vi "pulse_generator_data_v3.vi"(3 "Pulse Generator Offsets & Data Saving Controls":T3={"PG-TS Offset"=11500.0, "Pitot Offset"=0.0, "PG Abs Offset"=11500.0, "Sampling\nFrequency"=1000.0, "Recording Duration"=10.0}, 4 "PG Data":waveform(dbl)[](array[waveform]), 5 "Session Start Time":timestamp) -> (0 "Pulse Generator Charts":T1={" Camera Voltage"=9.650720988784618, "Pitot dP"=-0.0006103608758678569, "Absolute Tank Pressure"=119484.80284900061, "Pulse Generator to Test Section dP"=11360.460004869077}, 1 "Pulse Generator Measurements":T2={"PG to TS dP"=4351.8068090218785, "PG Abs"=119484.80284900061, "Mass Flow Rate"=nan, "Pitot dP"=-4308.9404273994505, "Pitot Amps"=2.6415199999999147e-07, "Vapor Temperature"=19.805676371442082, "Liquid Temperature"=19.52526901660894, "Vapor Sat Pressure"=121.24568157832624, "Liquid Sat Pressure"=119.96937909943745, "W1-4 dP[Pa]"=19.52526901660894, "W1-7 dP[Pa]"=119.96937909943745}, 2 "PG Data - Queue":dbl[][](array[numeric]))   [LabVIEW 2016]
uses:
  Sensor Translation/sensor_translation.lvlib
  Sensor Translation/Pressure Transducers/Omega/omega_px209_060a5v.vi
  pulse_generator_data.ctl
  <vilib>/Waveform/WDTOps.llb/WDT Get Waveform Time Array DBL.vi
  pulse_generator_data_charts.ctl
  pulse_generator_data_controls.ctl
panel:
  # "Pulse Generator - Test Section dP"
  # "Pulse Generator Absolute Pressure"
  # "Pitot dP"
  # "Pitot Current"
  # "Mass Flow Rate"
  # "Offsets"
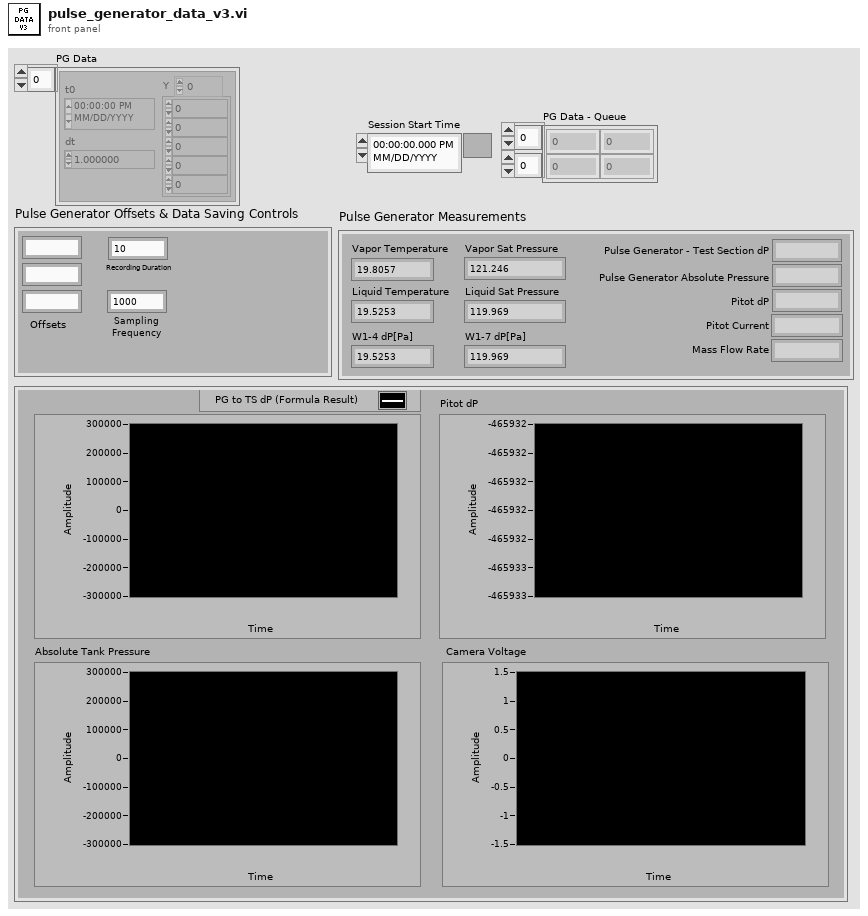
[diagram p1: front panel]
types:
  T1 = typedef "pulse_generator_data_charts.ctl" = cluster{" Camera Voltage":dbl, "Pitot dP":dbl, "Absolute Tank Pressure":dbl, "Pulse Generator to Test Section dP":dbl}
  T2 = typedef "pulse_generator_data.ctl" = cluster{"PG to TS dP":dbl, "PG Abs":dbl, "Mass Flow Rate":dbl, "Pitot dP":dbl, "Pitot Amps":dbl, "Vapor Temperature":dbl, "Liquid Temperature":dbl, "Vapor Sat Pressure":dbl, "Liquid Sat Pressure":dbl, "W1-4 dP[Pa]":dbl, "W1-7 dP[Pa]":dbl}
  T3 = typedef "pulse_generator_data_controls.ctl" = cluster{"PG-TS Offset":dbl, "Pitot Offset":dbl, "PG Abs Offset":dbl, "Sampling\nFrequency":dbl, "Recording Duration":dbl}
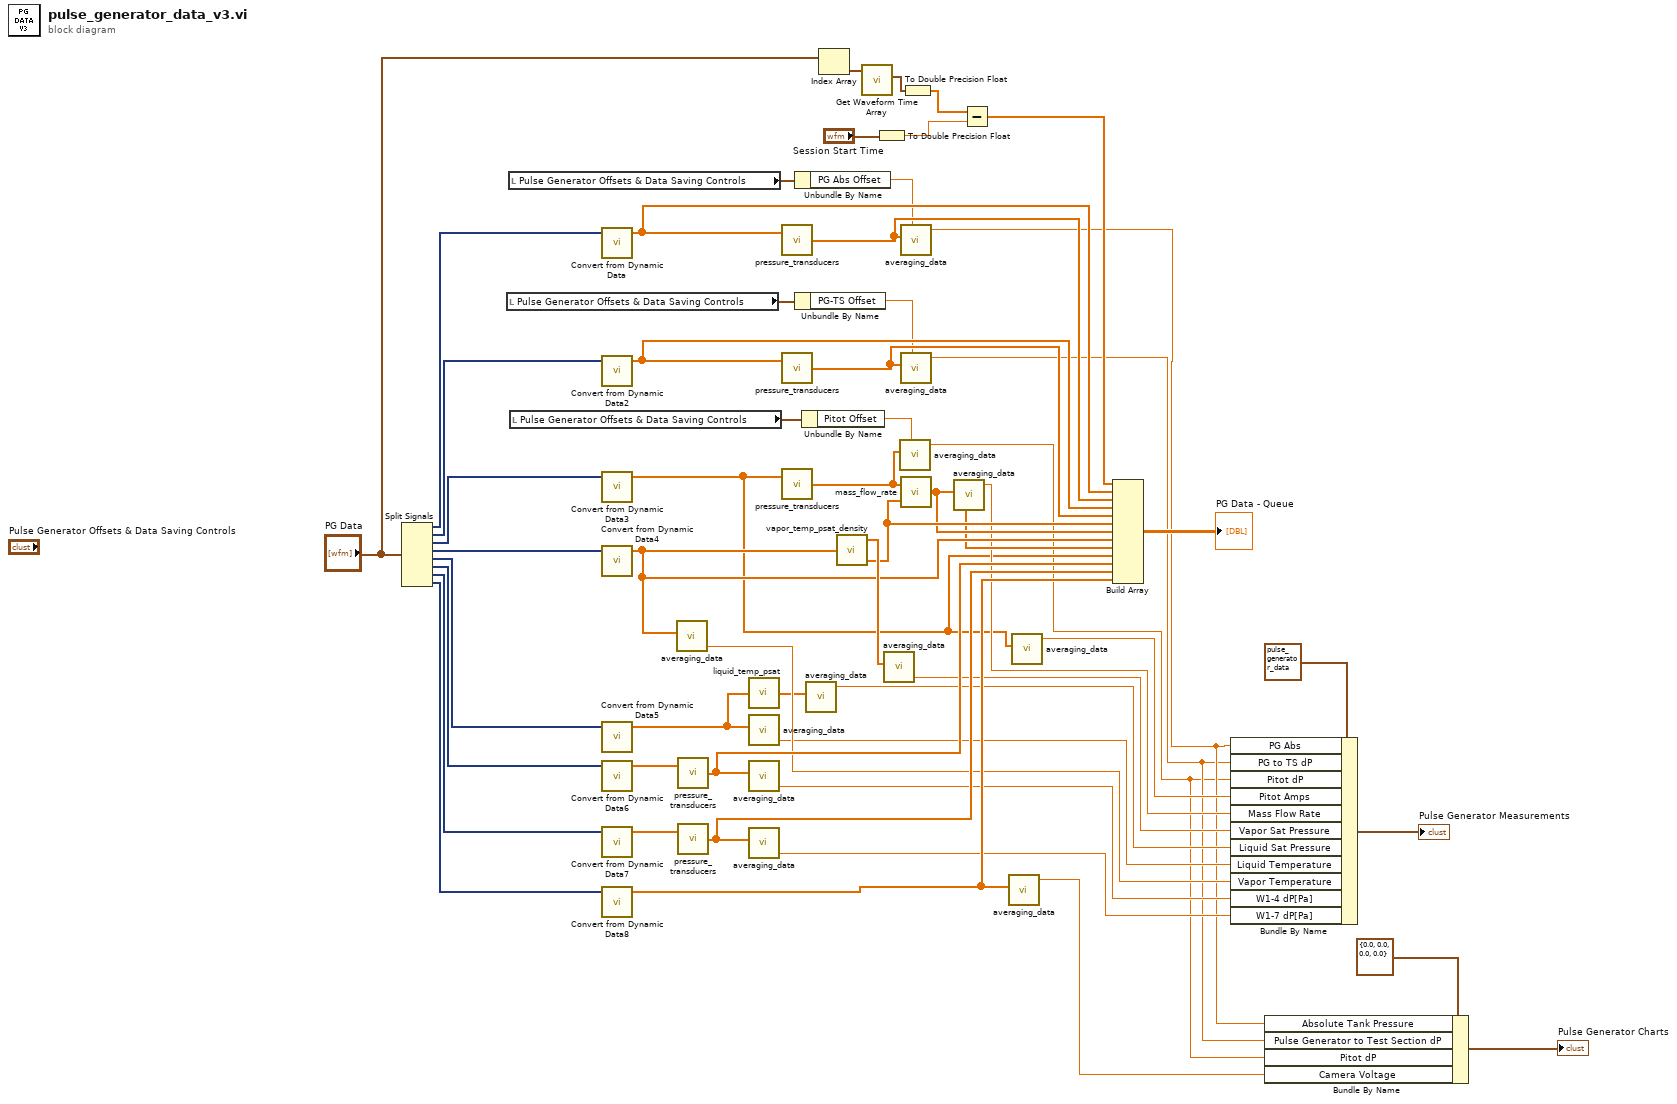
[diagram p0: block diagram]
diagram:
  n1 = Split Signals("PG Data") -> (w37:dynamicdata, w36:dynamicdata, w56:dynamicdata, w55:dynamicdata, w53:dynamicdata, w52:dynamicdata, w50:dynamicdata, w48:dynamicdata)  [unwired: 8 in]
  n2 = local read "Pulse Generator Offsets & Data Saving Controls"() -> (w24:T3)
  n3 = local read "Pulse Generator Offsets & Data Saving Controls"() -> (w26:T3)
  n4 = local read "Pulse Generator Offsets & Data Saving Controls"() -> (w22:T3)
  n5 = call "Convert from Dynamic Data"("Dynamic Data Type"=w37) -> ("Array"=w33:dbl[])  [unwired: 3 in]
  n6 = call "Convert from Dynamic Data2"("Dynamic Data Type"=w36) -> ("Array"=w34:dbl[])  [unwired: 3 in]
  n7 = call "Convert from Dynamic Data3"("Dynamic Data Type"=w56) -> ("Array"=w9:dbl[])  [unwired: 3 in]
  n8 = call "Convert from Dynamic Data4"("Dynamic Data Type"=w55) -> ("Array"=w32:dbl[])  [unwired: 3 in]
  n9 = call "Convert from Dynamic Data5"("Dynamic Data Type"=w53) -> ("Array"=w14:dbl[])  [unwired: 3 in]
  n10 = call "Convert from Dynamic Data6"("Dynamic Data Type"=w52) -> ("Array"=w51:dbl[])  [unwired: 3 in]
  n11 = call "Convert from Dynamic Data7"("Dynamic Data Type"=w50) -> ("Array"=w49:dbl[])  [unwired: 3 in]
  n12 = call "Convert from Dynamic Data8"("Dynamic Data Type"=w48) -> ("Array"=w28:dbl[])  [unwired: 3 in]
  n13 = call "averaging_data.vi"("Input"=w32) -> ("Offset Average"=w16:dbl)  [unwired: 5 in, 2 out]
  n14 = call-poly "pressure_transducers.vi"("Source"=w51) -> ("Target"=w30:dbl[])  [unwired: 1 in]
  n15 = call-poly "pressure_transducers.vi"("Source"=w49) -> ("Target"=w29:dbl[])  [unwired: 1 in]
  n16 = call "liquid_temp_psat.vi"("Liquid Temp [C]"=w14) -> ("Psat Liquid"=w13:dbl[])
  n17 = call "averaging_data.vi"("Input"=w14) -> ("Offset Average"=w15:dbl)  [unwired: 5 in, 2 out]
  n18 = call "averaging_data.vi"("Input"=w30) -> ("Offset Average"=w17:dbl)  [unwired: 5 in, 2 out]
  n19 = call "averaging_data.vi"("Input"=w29) -> ("Offset Average"=w18:dbl)  [unwired: 5 in, 2 out]
  n20 = call-poly "pressure_transducers.vi"("Source"=w33) -> ("Target"=w40:dbl[])  [unwired: 1 in]
  n21 = call-poly "pressure_transducers.vi"("Source"=w34) -> ("Target"=w39:dbl[])  [unwired: 1 in]
  n22 = call-poly "pressure_transducers.vi"("Source"=w9) -> ("Target"=w27:dbl[])  [unwired: 1 in]
  n23 = Unbundle By Name(w26) -> ("PG Abs Offset"=w25:dbl)
  n24 = Unbundle By Name(w24) -> ("PG-TS Offset"=w23:dbl)
  n25 = Unbundle By Name(w22) -> ("Pitot Offset"=w21:dbl)
  n26 = call "averaging_data.vi"("Input"=w13) -> ("Average"=w11:dbl)  [unwired: 5 in, 2 out]
  n27 = Index Array(array="PG Data") -> (element=w47:waveform(dbl))  [unwired: 1 in]
  n28 = call "vapor_temp_psat_density.vi"("Vapor Temp [C]"=w32) -> ("Psat Vapor"=w54:dbl[], "Vapor Density"=w38:dbl[])  [unwired: 1 in]
  n29 = call-poly <vilib>:"Get Waveform Time Array.vi"("waveform in"=w47) -> ("X array"=w46:timestamp[])  [unwired: 9 in, 1 out]
  n30 = To Double Precision Float(number="Session Start Time") -> (double precision float=w43:dbl)
  n31 = call "averaging_data.vi"("Input"=w54) -> ("Offset Average"=w12:dbl)  [unwired: 5 in, 2 out]
  n32 = call "averaging_data.vi"("Offset"=w21, "Input"=w27) -> ("Average"=w2:dbl)  [unwired: 4 in, 2 out]
  n33 = call "averaging_data.vi"("Offset"=w25, "Input"=w40) -> ("Average"=w4:dbl)  [unwired: 4 in, 2 out]
  n34 = call "averaging_data.vi"("Offset"=w23, "Input"=w39) -> ("Average"=w3:dbl)  [unwired: 4 in, 2 out]
  n35 = call "mass_flow_rate.vi"("Density"=w38, "dP H2O"=w27) -> ("Mass Flow Rate [g/s] Array"=w35:dbl[])
  n36 = To Double Precision Float(number=w46) -> (double precision float=w42:dbl[])
  n37 = call "averaging_data.vi"("Input"=w35) -> ("Input Offset"=w31:dbl[], "Average"=w10:dbl)  [unwired: 5 in, 1 out]
  n38 = Subtract(x=w42, y=w43) -> (x-y=w41:dbl[])
  n39 = call "averaging_data.vi"("Input"=w28) -> ("Average"=w1:dbl)  [unwired: 5 in, 2 out]
  n40 = call "averaging_data.vi"("Input"=w9) -> ("Average"=w8:dbl)  [unwired: 5 in, 2 out]
  n41 = Build Array(w41, w33, w40, w34, w39, w38, w35, w32, w31, w9, w30, w29, w28) -> (→"PG Data - Queue":dbl[][])
  n42 = Bundle By Name(cluster=T2 {"PG to TS dP"=4351.8068090218785, "PG Abs"=119484.80284900061, "Mass Flow Rate"=nan, "Pitot dP"=-4308.9404273994505, "Pitot Amps"=2.6415199999999147e-07, "Vapor Temperature"=19.805676371442082, "Liquid Temperature"=19.52526901660894, "Vapor Sat Pressure"=121.24568157832624, "Liquid Sat Pressure"=119.96937909943745, "W1-4 dP[Pa]"=19.52526901660894, "W1-7 dP[Pa]"=119.96937909943745} ("Pulse Generator Measurements"), "PG Abs"=w4, "PG to TS dP"=w3, "Pitot dP"=w2, "Pitot Amps"=w8, "Mass Flow Rate"=w10, "Vapor Sat Pressure"=w12, "Liquid Sat Pressure"=w11, "Liquid Temperature"=w15, "Vapor Temperature"=w16, "W1-4 dP[Pa]"=w17, "W1-7 dP[Pa]"=w18) -> (→"Pulse Generator Measurements":T2)
  n43 = Bundle By Name(cluster=T1 {" Camera Voltage"=0.0, "Pitot dP"=0.0, "Absolute Tank Pressure"=0.0, "Pulse Generator to Test Section dP"=0.0} ("Pulse Generator Charts 2"), "Absolute Tank Pressure"=w4, "Pulse Generator to Test Section dP"=w3, "Pitot dP"=w2, "Camera Voltage"=w1) -> (→"Pulse Generator Charts":T1)
